vi "Reanimate.vi"(6 "Variant in":variant, 7 "Shift Pressed?":bool, 8 "error in (no error)":errorcluster, 10 "QD Combo Box Ref":refnum<vi>, 11 "QD Launch VI Ref":refnum<vi>) -> (0 "error out":errorcluster, 4 "Variant out":variant)   [LabVIEW 2017, in "Quick Drop.lvlib"]
doc: "Reanimates a corpse at a grave. The Spirit frame (new, refactored code) is disabled and the Corpse frame (legacy code) is enabled for the grave (Diagram Disable structure), but the \"Corpse\" subdiagram label is changed to a \"Zombie\" label because the legacy code has been brought back from the dead. A timestamp is included in the \"Zombie\" label that indicates the last time the legacy code was used. The date is automatically set to the date when the corpse is revived.\n\nDefault Shortcut - [Z]"
uses:
  Quick Drop.lvlib
  Toolkit VIs/Toolkit.lvlib
panel:
  in  "Undo Name":string="Reanimate"
  # "Do not change the connector pane of this VI.\n\nSee the block diagram for directions on how to use this template."
  # "Specify the name of the Undo transaction"
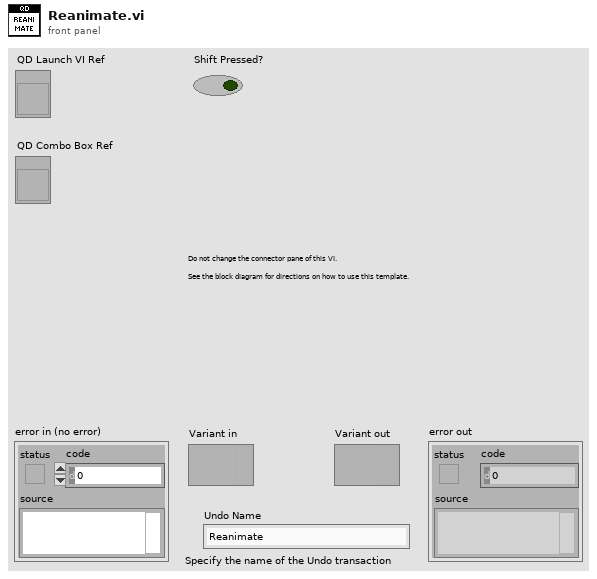
[diagram p1: front panel]
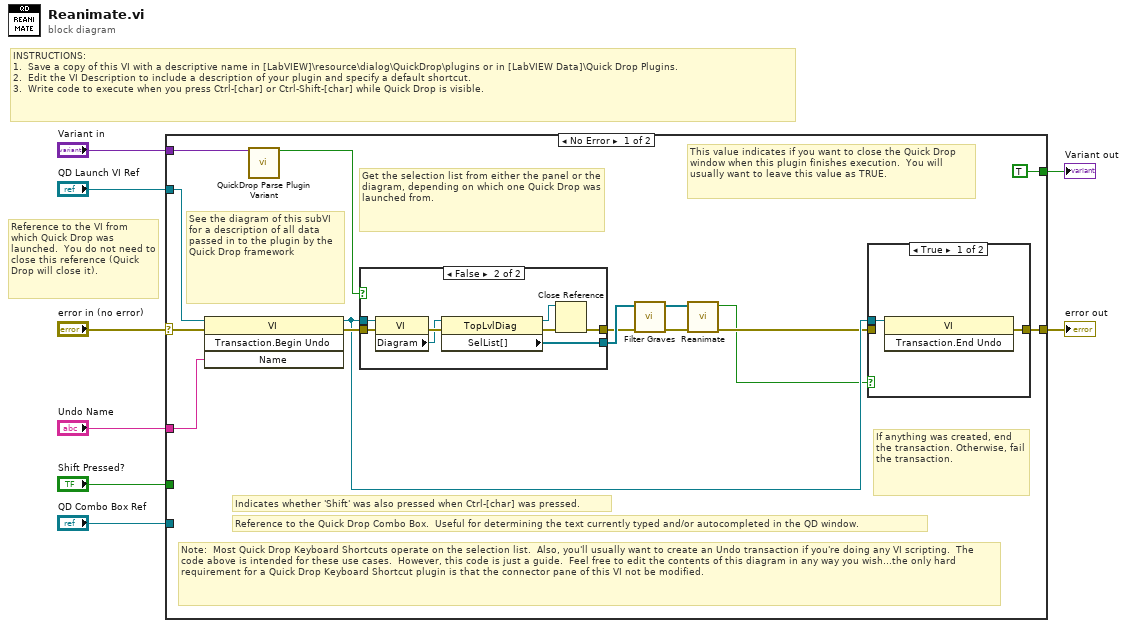
[diagram p0: block diagram]
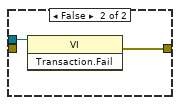
[diagram p2: hidden frame]
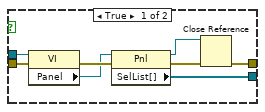
[diagram p3: hidden frame]
diagram:
  # "Reference to the VI from which Quick Drop was launched.  You do not need to close this reference (Quick Drop will close it)."
  # "INSTRUCTIONS:\n1.  Save a copy of this VI with a descriptive name in [LabVIEW]\\resource\\dialog\\QuickDrop\\plugins or in [LabVIEW Data]\\Quick Drop Plugins.\n2.  Edit the VI Description to include a description of your plugin and specify a default shortcut. \n3.  Write code to execute when you press Ctrl-[char] or Ctrl-Shift-[char] while Quick Drop is visible."
  n1 = case shown="No Error" "error in (no error)" {
    selector: "error in (no error)" -> [w22 w44]
    tunnel: [w16 w44] -> w7
    tunnel: "QD Launch VI Ref" -> [w21 _]
    tunnel: "Shift Pressed?" -> [_ _]
    tunnel: "QD Combo Box Ref" -> [_ _]
    tunnel: "Variant in" -> [w23 _]
    tunnel: "Undo Name" -> [w20 _]
    tunnel: [TRUE _] -> w1
    frame No Error {
      # "Note:  Most Quick Drop Keyboard Shortcuts operate on the selection list.  Also, you'll usually want to create an Undo transaction if you're doing any VI scripting.  The code above is intended for these use cases.  However, this code is just a guide.  Feel free to edit the contents of this diagram in any way you wish...the only hard requirement for a Quick Drop Keyboard Shortcut plugin is that the connector pane of this VI not be modified."
      # "Get the selection list from either the panel or the diagram, depending on which one Quick Drop was launched from."
      # "If anything was created, end the transaction. Otherwise, fail the transaction."
      # "This value indicates if you want to close the Quick Drop window when this plugin finishes execution.  You will usually want to leave this value as TRUE."
      # "See the diagram of this subVI for a description of all data passed in to the plugin by the Quick Drop framework"
      # "Reference to the Quick Drop Combo Box.  Useful for determining the text currently typed and/or autocompleted in the QD window."
      # "Indicates whether 'Shift' was also pressed when Ctrl-[char] was pressed."
      n2 = invoke class="VI" method="Transaction.Begin Undo"(reference=w21, error in=w22, "Name"=w20) -> (reference out=w15:refnum<vi>, error out=w17:errorcluster)  [unwired: 1 in, 2 out]
      n3 = call <vilib>:"QuickDrop Parse Plugin Variant.vi"("QDKS Variant in"=w23) -> ("QD Launch VI Panel?"=w18:bool)  [unwired: 12 in, 2 out]
      n4 = case shown="False" w18 {
        tunnel: w17 -> [w35 w43]
        tunnel: w15 -> [w34 w42]
        tunnel: [w29 w37] -> w11
        tunnel: [w28 w36] -> w12
        frame True {
          n5 = property class="VI"(reference=w34, error in=w35) -> (error out=w33:errorcluster, "Panel"=w32:refnum<vi>)  [unwired: 1 out]
          n6 = property class="Pnl"(reference=w32, error in=w33) -> (reference out=w30:refnum<vi>, error out=w31:errorcluster, "SelList[]"=w28:refnum<vi>[])
          n7 = Close Reference(reference=w30, error in (no error)=w31) -> (error out=w29:errorcluster)
        }
        frame False {
          n8 = property class="VI"(reference=w42, error in=w43) -> (error out=w41:errorcluster, "Diagram"=w40:refnum<vi>)  [unwired: 1 out]
          n9 = property class="TopLvlDiag"(reference=w40, error in=w41) -> (reference out=w38:refnum<vi>, error out=w39:errorcluster, "SelList[]"=w36:refnum<vi>[])
          n10 = Close Reference(reference=w38, error in (no error)=w39) -> (error out=w37:errorcluster)
        }
      }
      n11 = call "Filter Graves.vi"("Error In"=w11, "GObjects"=w12) -> ("Error Out"=w10:errorcluster, "Graves"=w9:refnum<vi>[])  [unwired: 8 in]
      n12 = call "Reanimate.vi"("Error In"=w10, "Graves"=w9) -> ("Error Out"=w14:errorcluster, "Change Made?"=w13:bool)  [unwired: 8 in]
      n13 = case shown="True" w13 {
        tunnel: w15 -> [w24 w26]
        tunnel: [w25 w27] -> w16
        tunnel: w14 -> [_ _]
        frame True {
          n14 = invoke class="VI" method="Transaction.End Undo"(reference=w24) -> (error out=w25:errorcluster)  [unwired: 2 in, 2 out]
        }
        frame False {
          n15 = invoke class="VI" method="Transaction.Fail"(reference=w26) -> (error out=w27:errorcluster)  [unwired: 2 in, 2 out]
        }
      }
    }
    frame Error {
    }
  }
  "error out" <- w7
  "Variant out" <- w1
